vi "Generate SVG Attribute Object.vi"(8 "error in (no error)":errorcluster, 11 "Named Cluster of Data":variant) -> (0 "error out":errorcluster, 3 "SVG Attribute Object":string)   [LabVIEW 2019, in "EditSVG.lvclass"]
uses:
  EditSVG.lvclass
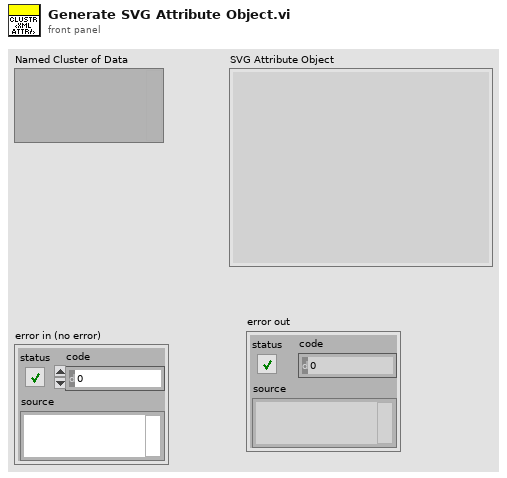
[diagram p1: front panel]
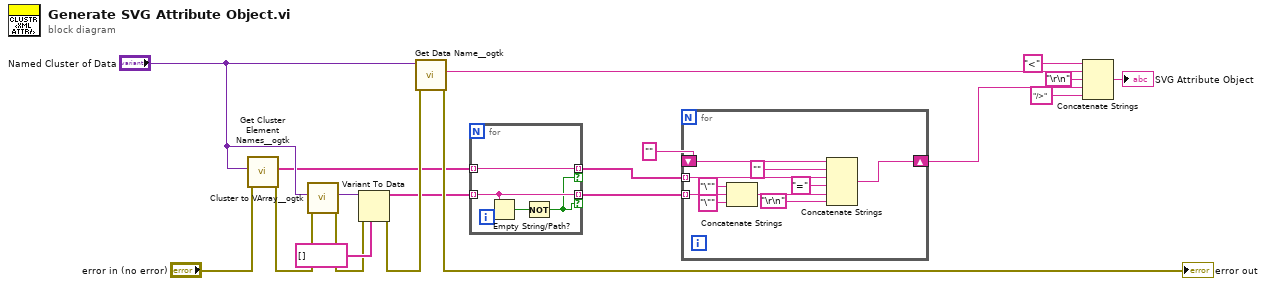
[diagram p0: block diagram]
diagram:
  n1 = call <userlib>:"Get Cluster Element Names__ogtk.vi"("error in (no error)"="error in (no error)", "Cluster"="Named Cluster of Data") -> ("error out"=w8:errorcluster, "Element Names"=w4:string[])  [unwired: 8 in]
  n2 = call <userlib>:"Cluster to VArray__ogtk.vi"("error in (no error)"=w8, "Cluster"="Named Cluster of Data") -> ("error out"=w9:errorcluster, "VArray"=w19:variant)  [unwired: 8 in]
  n3 = Variant To Data(error in=w9, type=string[] [], Variant=w19) -> (data=w3:string[], error out=w10:errorcluster)
  n4 = call <userlib>:"Get Data Name__ogtk.vi"("error in (no error)"=w10, "Data"="Named Cluster of Data") -> ("error out"=→"error out":errorcluster, "Data Name"=w13:string)  [unwired: 7 in, 1 out]
  n5 = for {
    tunnel: w4 -> [w21] mode=indexing
    tunnel: w3 -> [w22] mode=indexing
    tunnel: [w22] -> w2 mode=indexing if=w20
    tunnel: [w21] -> w1 mode=indexing if=w20
    n6 = Empty String/Path?(string/path=w22) -> (empty?=w23:bool)
    n7 = Not(x=w23) -> (.not. x?=w20:bool)
  }
  n8 = for {
    shift-right: [w26] -> w15
    shift-left: "" -> [w25]
    tunnel: w1 -> [w33] mode=indexing
    tunnel: w2 -> [w31] mode=indexing
    n9 = Concatenate Strings("\"" ("string"), w31, "\"" ("string")) -> (w28:string)
    n10 = Concatenate Strings(w25, "" ("string"), w33, "=" ("string"), w28, "\r\n") -> (w26:string)
  }
  n11 = Concatenate Strings("<", w13, "\r\n", w15, "/>" ("string")) -> (→"SVG Attribute Object":string)
